vi "Notebook.vi"() -> ()   [LabVIEW 2019, in "Notebook.lvlib"]
uses:
  Notebook.lvlib
  System.Windows.Forms
  Notebook Action Q Element.ctl
  Notebook Action List.ctl
  System.Drawing
  Rich Text Box/Text Colors.ctl
  Rich Text Box/Formatted Text.ctl
  Rich Text Box/Text Formatting.ctl
  Notebook Saved Global.vi
  Rich Text Box/Rich Text Box.lvlib
  Variant/Variant to Data/Variant to Data.lvlib
panel:
  in  "Notebook Content":refnum<k24>(container)
types:
  T1 = enum32{"Invalid", "Standard", "Closed", "Hidden", "Minimized", "Maximized"}
  T2 = typedef "Notebook.lvlib/Notebook Action Q Element.ctl" = cluster{"Action":T3, "Variant":variant}
  T3 = typedef "Notebook.lvlib/Notebook Action List.ctl" = enum16{"Idle", "Init", "Check Content Change", "User added content", "Program added text", "Program added Picture ", "Save Notebook", "Quit", "Open", "Close", "Update Window Title"}
  T4 = typedef "Rich Text Box.lvlib/Text Colors.ctl" = enum16{"Unchanged", "Black", "Blue", "Gray", "Green", "Red", "White"}
  T5 = typedef "Rich Text Box.lvlib/Formatted Text.ctl" = cluster{"Text":string, "Text Formatting":T6}
  T6 = typedef "Rich Text Box.lvlib/Text Formatting.ctl" = cluster{"Font":string, "Text Color":T4, "Text Background Color":T4, "Text Style":enum16{"Regular", "Bold", "Italic", "Underline", "Strikeout"}, "Font Size (Points)":dbl, "Text Alignment":i32}
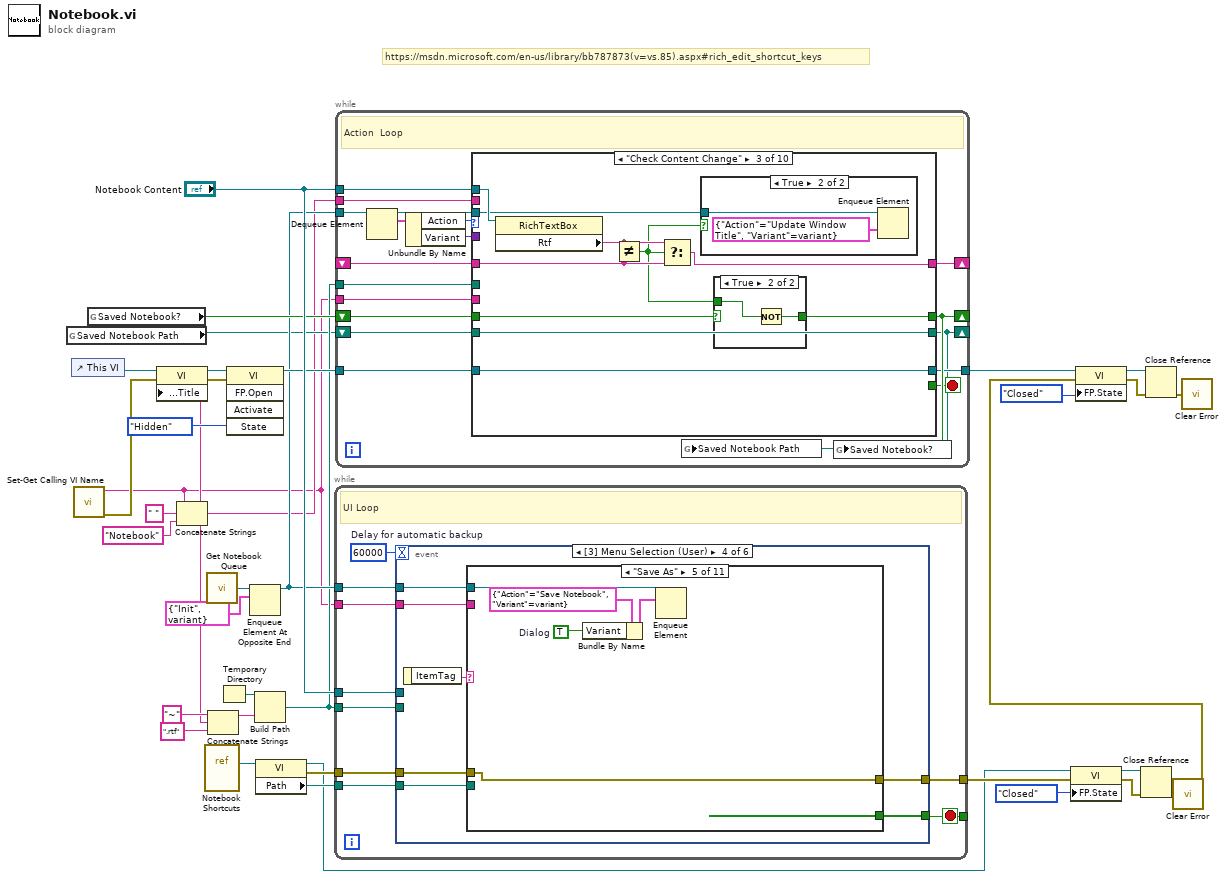
[diagram p0: block diagram]
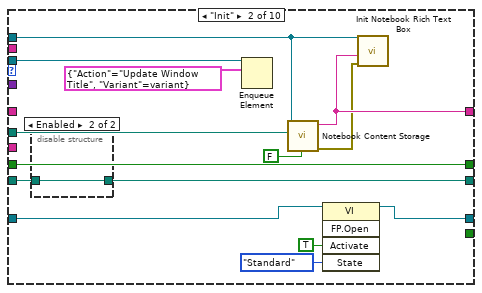
[diagram p3: hidden frame]
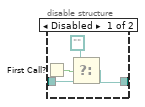
[diagram p4: hidden frame]
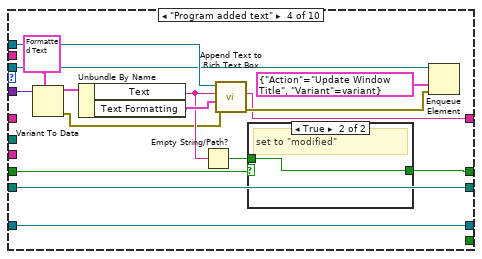
[diagram p7: hidden frame]
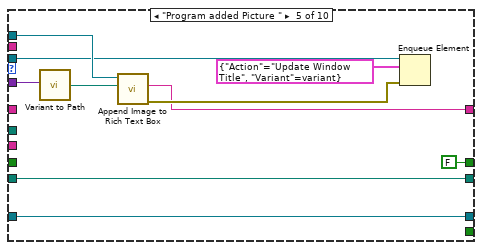
[diagram p9: hidden frame]
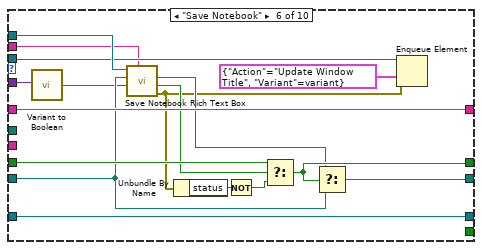
[diagram p10: hidden frame]
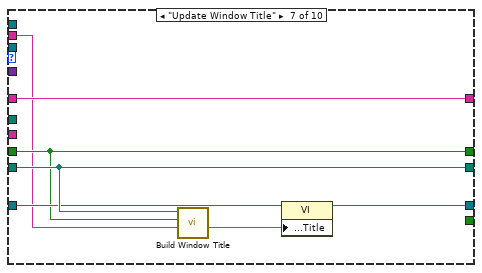
[diagram p11: hidden frame]
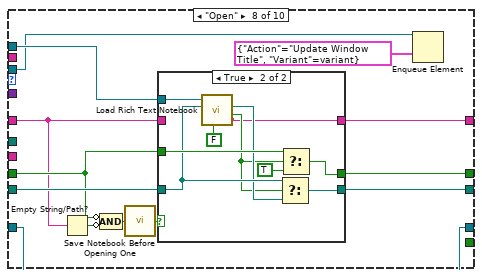
[diagram p12: hidden frame]
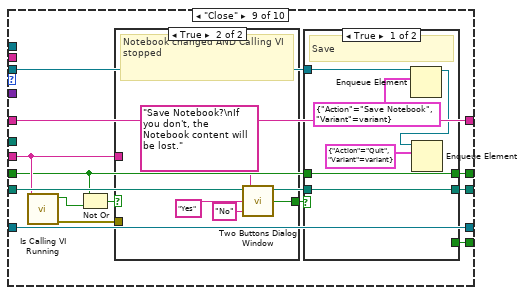
[diagram p14: hidden frame]
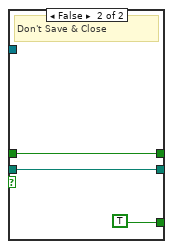
[diagram p15: hidden frame]
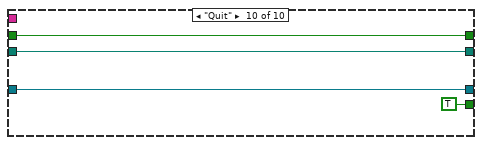
[diagram p17: hidden frame]
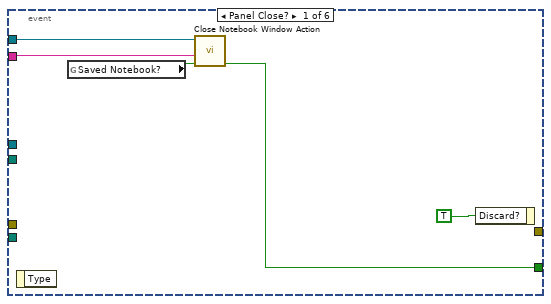
[diagram p18: hidden frame]
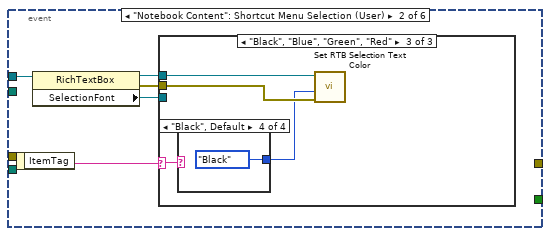
[diagram p19: hidden frame]
diagram:
  # "https://msdn.microsoft.com/en-us/library/bb787873(v=vs.85).aspx#rich_edit_shortcut_keys"
  n1 = global read "Notebook Saved Global.vi" "Saved Notebook Path"() -> (w17:path)
  n2 = control-ref of="This VI"() -> (w31:refnum<vi>)
  n3 = call "Set-Get Calling VI Name.vi"() -> ("Error Out"=w3:errorcluster, "Calling VI Name"=w1:string)  [unwired: 10 in]
  n4 = global read "Notebook Saved Global.vi" "Saved Notebook?"() -> (w28:bool)
  n5 = Concatenate Strings(w1, " " ("string"), "Notebook" ("string")) -> (w2:string)
  n6 = property class="VI"(reference=w31, error in=w3, "Front Panel.Title"=w2) -> (reference out=w25:refnum<vi>, error out=w16:errorcluster)
  n7 = vi-ref "Notebook Shortcuts.vi"() -> (w13:refnum<vi>)
  n8 = call "Get Notebook Queue.vi"() -> ("Notebook Queue"=w27:refnum<queue>)  [unwired: 9 in]
  n9 = Concatenate Strings("~" ("string"), w2, ".rtf" ("format string")) -> (w19:string)
  n10 = Temporary Directory() -> (w32:path)
  n11 = invoke class="VI" method="FP.Open"(reference=w25, error in=w16, "State"=T1."Hidden") -> (reference out=w30:refnum<vi>)  [unwired: 2 in, 4 out]
  n12 = Enqueue Element At Opposite End(queue=w27, element=T2 {"Action"=enum."Init", "Variant"=variant}) -> (queue out=w26:refnum<queue>)  [unwired: 2 in, 2 out]
  n13 = Build Path(base path=w32, name or relative path=w19) -> (appended path=w18:path)
  n14 = property class="VI"(reference=w13) -> (reference out=w7:refnum<vi>, error out=w12:errorcluster, "Path"=w11:path)  [unwired: 1 in]
  n15 = while {
    tunnel: w26 -> [w45]
    tunnel: "Notebook Content" -> [w43]
    tunnel: w1 -> [w41]
    tunnel: w18 -> [w42]
    tunnel: w12 -> [w40]
    tunnel: w11 -> [w39]
    tunnel: [w38] -> _
    tunnel: [w37] -> w8
    stop <- w38 stop-if-true
    w44 = 60000  # Delay for automatic backup
    # "UI Loop"
    n16 = event shown="[3] Menu Selection (User)" {
      selector: _ -> [_ _ _ _ _ _]
      dyn-events: _ -> [_ _ _ _ _ _]
      timeout: w44 -> [_ _ _ _ _ _]
      tunnel: [w49 _ _ w88 w129 _] -> w38
      tunnel: w45 -> [w50 _ w83 w89 w130 _]
      tunnel: w43 -> [_ w54 w81 _ _ w143]
      tunnel: w42 -> [_ _ w80 _ _ _]
      tunnel: w41 -> [w46 _ _ w87 w128 _]
      tunnel: w40 -> [_ _ _ w86 _ _]
      tunnel: w39 -> [_ _ _ w85 _ _]
      tunnel: [_ _ _ w84 _ _] -> w37
      event Panel Close? {
        n17 = event-data() -> ()  [unwired: 1 in, 1 out]
        n18 = global read "Notebook Saved Global.vi" "Saved Notebook?"() -> (w47:bool)
        n19 = call "Close Notebook Window Action.vi"("Notebook Saved?"=w47, "Main VI Name"=w46, "Notebook Queue"=w50) -> ("Quit?"=w49:bool)  [unwired: 8 in]
        n20 = event-data("Discard?"=TRUE) -> ()  [unwired: 1 in, 1 out]
      }
      event "Notebook Content": Shortcut Menu Selection (User) {
        n21 = event-data() -> ("ItemTag"=w55:string)  [unwired: 1 in]
        n22 = property class="RichTextBox"(reference=w54) -> (reference out=w51:refnum<k24>, error out=w52:errorcluster, "SelectionFont"=w53:refnum<k24>)  [unwired: 1 in]
        n23 = case shown="\"Black\", \"Blue\", \"Green\", \"Red\"" w55 {
          selector: w55 -> [_ w61 w72]
          tunnel: w53 -> [_ w65 _]
          tunnel: w52 -> [_ w60 w73]
          tunnel: w51 -> [_ w57 w74]
          frame "", Default {
          }
          frame "Bold", "Italic", "Regular", "Strikeout", "Underline" {
            n24 = property class="Font"(reference=w65, error in=w60) -> (error out=w59:errorcluster, "Name"=w64:string, "SizeInPoints"=w63:sgl)  [unwired: 1 out]
            n25 = case shown="\"Bold\"" w61 {
              tunnel: [w66 w67 w68 w69 w70] -> w62
              frame "Regular", Default {
                w66 = 0 items=["Regular"=0, "Bold"=1, "Italic"=2, "Underline"=4, "Strikeout"=8] ("style")
              }
              frame "Bold" {
                w67 = 1 items=["Regular"=0, "Bold"=1, "Italic"=2, "Underline"=4, "Strikeout"=8] ("style")
              }
              frame "Italic" {
                w68 = 2 items=["Regular"=0, "Bold"=1, "Italic"=2, "Underline"=4, "Strikeout"=8] ("style")
              }
              frame "Underline" {
                w69 = 4 items=["Regular"=0, "Bold"=1, "Italic"=2, "Underline"=4, "Strikeout"=8] ("style")
              }
              frame "Strikeout" {
                w70 = 8 items=["Regular"=0, "Bold"=1, "Italic"=2, "Underline"=4, "Strikeout"=8] ("style")
              }
            }
            n26 = constructor class="Font"(error in=w59, "familyName"=w64, "emSize"=w63, "unit"=w62) -> (reference out=w56:refnum<k24>, error out=w58:errorcluster)  [unwired: 2 in, 4 out]
            n27 = property class="RichTextBox"(reference=w57, error in=w58, "SelectionFont"=w56) -> ()  [unwired: 2 out]
          }
          frame "Black", "Blue", "Green", "Red" {
            n28 = case shown="\"Black\", Default" w72 {
              tunnel: [Text_Colors."Blue" ("Text Color") Text_Colors."Green" ("Text Color") Text_Colors."Red" ("Text Color") Text_Colors."Black" ("Text Color")] -> w71
              frame "Blue" {
              }
              frame "Green" {
              }
              frame "Red" {
              }
              frame "Black", Default {
              }
            }
            n29 = call "Set RTB Selection Text Color.vi"("Error In"=w73, "Text Color"=w71, ".NET RTB Refnum in"=w74) -> ()  [unwired: 7 in, 2 out]
          }
        }
      }
      event Timeout {
        n30 = event-data() -> ()  [unwired: 1 in, 1 out]
        n31 = call "Notebook Content Storage.vi"("Save(T)/Load(F)"=TRUE, "path"=w80, ".NET Refnum in"=w81) -> ()  [unwired: 7 in, 2 out]
        n32 = Enqueue Element(queue=w83, element=T2 {"Action"=enum."Check Content Change", "Variant"=variant}) -> ()  [unwired: 2 in, 3 out]
      }
      event Menu Selection (User) {
        n33 = event-data() -> ("ItemTag"=w90:string)  [unwired: 1 in]
        n34 = case shown="\"Save As\"" w90 {
          tunnel: w89 -> [_ _ w95 w100 w105 w110 _ w122 _ _ _]
          tunnel: [_ _ _ _ _ w109 _ _ _ _ _] -> w88
          tunnel: w87 -> [_ _ _ _ _ w107 _ _ _ _ _]
          tunnel: w86 -> [w91 w92 w93 w96 w101 w106 w111 w112 w123 w124 w126]
          tunnel: w85 -> [_ _ _ _ _ _ _ _ _ _ w127]
          tunnel: [w91 w92 w93 w96 w101 w106 w111 w112 w123 w124 w125] -> w84
          frame "", Default {
          }
          frame "---------File----------" {
          }
          frame "Open" {
            n35 = Enqueue Element(queue=w95, element=T2 {"Action"=enum."Open", "Variant"=variant}) -> ()  [unwired: 2 in, 3 out]
          }
          frame "Save" {
            w97 = FALSE  # No dialog
            n36 = Bundle By Name(cluster=T2 {"Action"=enum."Save Notebook", "Variant"=variant} ("element"), "Variant"=w97) -> (w98:T2)
            n37 = Enqueue Element(queue=w100, element=w98) -> ()  [unwired: 2 in, 3 out]
          }
          frame "Save As" {
            w102 = TRUE  # Dialog
            n38 = Bundle By Name(cluster=T2 {"Action"=enum."Save Notebook", "Variant"=variant} ("element"), "Variant"=w102) -> (w103:T2)
            n39 = Enqueue Element(queue=w105, element=w103) -> ()  [unwired: 2 in, 3 out]
          }
          frame "Close" {
            n40 = global read "Notebook Saved Global.vi" "Saved Notebook?"() -> (w108:bool)
            n41 = call "Close Notebook Window Action.vi"("Notebook Saved?"=w108, "Main VI Name"=w107, "Notebook Queue"=w110) -> ("Quit?"=w109:bool)  [unwired: 8 in]
          }
          frame "----------Edit----------" {
          }
          frame "Paste Current Date & Time" {
            n42 = call "Current Date & Time String.vi"() -> ("time string"=w113:string, "date string"=w114:string)  [unwired: 9 in, 1 out]
            n43 = Format Into String(format string="Current Date & Time: %s, %s" ("initial string"), w114, w113) -> (resulting string=w117:string)  [unwired: 2 in, 1 out]
            n44 = call "Message Style.vi"() -> ("Message Formatting"=w116:T6)
            n45 = Bundle By Name(cluster=T5 {"Text"="", "Text Formatting"={"Font"="Default", "Text Color"=enum."Unchanged", "Text Background Color"=enum."Unchanged", "Text Style"=enum."Regular", "Font Size (Points)"=-1.0, "Text Alignment"=0}} ("Formatted Text"), "Text"=w117, "Text Formatting"=w116) -> (w118:T5)
            n46 = Bundle By Name(cluster=T2 {"Action"=enum."Program added text", "Variant"=variant} ("element"), "Variant"=w118) -> (w120:T2)
            n47 = Enqueue Element(queue=w122, element=w120) -> ()  [unwired: 2 in, 3 out]
          }
          frame "Find..." {
          }
          frame "-------- Help ---------" {
          }
          frame "Show Notebook Shortcuts" {
            n48 = call "Run Vi.vi"("VI Path"=w127, "error in (no error)"=w126) -> ("error out"=w125:errorcluster)  [unwired: 6 in, 1 out]
          }
        }
      }
      event "Notebook Content": Shortcut Menu Selection (App) {
        n49 = event-data() -> ("ItemTag"=w131:string)  [unwired: 1 in, 1 out]
        n50 = case shown="\"Paste Current Date & Time\"" w131 {
          tunnel: w130 -> [_ w142]
          tunnel: [_ FALSE ("Quit?")] -> w129
          tunnel: w128 -> [_ _]
          frame "", Default {
          }
          frame "Paste Current Date & Time" {
            n51 = call "Current Date & Time String.vi"() -> ("time string"=w134:string, "date string"=w133:string)  [unwired: 9 in, 1 out]
            n52 = Format Into String(format string="Current Date & Time: %s, %s" ("initial string"), w133, w134) -> (resulting string=w137:string)  [unwired: 2 in, 1 out]
            n53 = call "Message Style.vi"() -> ("Message Formatting"=w136:T6)
            n54 = Bundle By Name(cluster=T5 {"Text"="", "Text Formatting"={"Font"="Default", "Text Color"=enum."Unchanged", "Text Background Color"=enum."Unchanged", "Text Style"=enum."Regular", "Font Size (Points)"=-1.0, "Text Alignment"=0}} ("Formatted Text"), "Text"=w137, "Text Formatting"=w136) -> (w138:T5)
            n55 = Bundle By Name(cluster=T2 {"Action"=enum."Program added text", "Variant"=variant} ("element"), "Variant"=w138) -> (w140:T2)
            n56 = Enqueue Element(queue=w142, element=w140) -> ()  [unwired: 2 in, 3 out]
          }
        }
      }
      event Panel Resize {
        n57 = event-data() -> ()  [unwired: 1 in, 1 out]
        n58 = disable-structure shown="Enabled" {
          disable-tunnel: w143 -> [_ w145]
          frame Disabled {
            w144 = inf
          }
          frame Enabled {
            n59 = invoke class="RichTextBox" method="ScrollToCaret"(reference=w145) -> ()  [unwired: 2 in, 3 out]
          }
        }
      }
    }
  }
  n60 = while {
    tunnel: w26 -> [w163]
    shift-right: [w156] -> _
    shift-left: w28 -> [w160]
    shift-right: [w147] -> _
    shift-left: w17 -> [w159]
    tunnel: w30 -> [w153]
    tunnel: [w151] -> w36
    tunnel: "Notebook Content" -> [w155]
    tunnel: w1 -> [w152]
    shift-right: [w150] -> _
    shift-left: _ -> [w149]
    tunnel: w18 -> [w148]
    tunnel: w2 -> [w146]
    stop <- w154 stop-if-true
    # "Action  Loop"
    n61 = Dequeue Element(queue=w163) -> (queue out=w158:refnum<queue>, element=w162:T2)  [unwired: 2 in, 2 out]
    n62 = Unbundle By Name(w162) -> ("Action"=w161:T3, "Variant"=w157:variant)
    n63 = case shown="\"Check Content Change\"" w161 {
      tunnel: w160 -> [w167 w168 w189 w204 _ w242 w249 w263 w282 w310]
      tunnel: [w167 w168 w188 w203 FALSE ("Saved?") w237 w249 w264 w291 w310] -> w156
      tunnel: w159 -> [w166 w178 w196 w217 w229 w239 w253 w266 w289 w309]
      tunnel: [w166 w177 w196 w217 w229 w240 w253 w265 w288 w309] -> w147
      tunnel: w158 -> [_ w170 w190 w206 w222 w236 _ w256 w290 _]
      tunnel: w157 -> [_ _ _ w215 w227 w234 _ _ _ _]
      tunnel: w155 -> [_ w172 w194 w216 w228 w246 _ w259 _ _]
      tunnel: [_ _ _ _ _ _ _ _ w287 TRUE] -> w154
      tunnel: w153 -> [w165 w181 w195 w209 w224 w243 w251 w258 w286 w307]
      tunnel: w152 -> [_ _ _ _ _ _ _ _ w284 _]
      tunnel: [w165 w176 w195 w209 w224 w243 w250 w258 w286 w307] -> w151
      tunnel: [w164 w175 w191 w205 w220 w241 w248 w255 w285 _] -> w150
      tunnel: w149 -> [w164 _ w192 _ _ w241 w248 w254 w285 _]
      tunnel: w148 -> [_ w173 _ _ _ _ _ _ _ _]
      tunnel: w146 -> [_ _ _ _ _ w230 w247 _ _ _]
      frame "Idle", Default {
      }
      frame "Init" {
        n64 = disable-structure shown="Enabled" {
          disable-tunnel: w178 -> [w185 w186]
          disable-tunnel: [w184 w186] -> w177
          frame Disabled {
            n65 = First Call?() -> (First Call?: T/F=w182:bool)
            n66 = Select(t=path "", s=w182, f=w185) -> (s? t:f=w184:path)
          }
          frame Enabled {
          }
        }
        n67 = Enqueue Element(queue=w170, element=T2 {"Action"=enum."Update Window Title", "Variant"=variant}) -> ()  [unwired: 2 in, 3 out]
        n68 = call "Notebook Content Storage.vi"("Save(T)/Load(F)"=FALSE ("Set(T)/Get(F)"), "path"=w173, ".NET Refnum in"=w172) -> ("Error Out"=w171:errorcluster, "RTF content"=w175:string)  [unwired: 7 in]
        n69 = invoke class="VI" method="FP.Open"(reference=w181, "Activate"=TRUE ("Activate?"), "State"=T1."Standard") -> (reference out=w176:refnum<vi>)  [unwired: 2 in, 4 out]
        n70 = call "Init Notebook Rich Text Box.vi"("Error In"=w171, "Notebook Content"=w175, ".NET Refnum in"=w172) -> ()  [unwired: 8 in, 1 out]
      }
      frame "Check Content Change" {
        n71 = property class="RichTextBox"(reference=w194) -> ("Rtf"=w193:string)  [unwired: 1 in, 2 out]
        n72 = Not Equal?(x=w193, y=w192) -> (x != y?=w187:bool)
        n73 = Select(t=w193, s=w187, f=w192) -> (s? t:f=w191:string)
        n74 = case shown="True" w187 {
          tunnel: w190 -> [_ w201]
          frame False {
          }
          frame True {
            n75 = Enqueue Element(queue=w201, element=T2 {"Action"=enum."Update Window Title", "Variant"=variant}) -> ()  [unwired: 2 in, 3 out]
          }
        }
        n76 = case shown="True" w189 {
          selector: w189 -> [w197 _]
          tunnel: [w197 w198] -> w188
          tunnel: w187 -> [_ w199]
          frame False {
          }
          frame True {
            n77 = Not(x=w199) -> (.not. x?=w198:bool)
          }
        }
      }
      frame "Program added text" {
        n78 = Variant To Data(type=T5 {"Text"="", "Text Formatting"={"Font"="Default", "Text Color"=enum."Unchanged", "Text Background Color"=enum."Unchanged", "Text Style"=enum."Regular", "Font Size (Points)"=-1.0, "Text Alignment"=0}} ("Formatted Text"), Variant=w215) -> (data=w213:T5, error out=w210:errorcluster)  [unwired: 1 in]
        n79 = Unbundle By Name(w213) -> ("Text"=w211:string, "Text Formatting"=w212:T6)
        n80 = Empty String/Path?(string/path=w211) -> (empty?=w202:bool)
        n81 = call "Append Text to Rich Text Box.vi"("error in (no error)"=w210, "Text Formatting"=w212, "String"=w211, ".NET Refnum in"=w216) -> ("Error Out"=w207:errorcluster, "Rtf Content"=w205:string)  [unwired: 6 in]
        n82 = case shown="True" w204 {
          selector: w204 -> [w218 _]
          tunnel: [w218 w219] -> w203
          tunnel: w202 -> [_ w219]
          frame False {
            # "remains \"modified\""
          }
          frame True {
            # "set to \"modified\""
          }
        }
        n83 = Enqueue Element(queue=w206, element=T2 {"Action"=enum."Update Window Title", "Variant"=variant}, error in (no error)=w207) -> ()  [unwired: 1 in, 3 out]
      }
      frame "Program added Picture " {
        n84 = call "Variant to Path.vi"("Variant"=w227) -> ("Path"=w226:path)  [unwired: 8 in]
        n85 = call "Append Image to Rich Text Box.vi"("Image File Path"=w226, ".NET Refnum in"=w228) -> ("error out"=w221:errorcluster, "Rtf Content"=w220:string)  [unwired: 8 in]
        n86 = Enqueue Element(queue=w222, element=T2 {"Action"=enum."Update Window Title", "Variant"=variant}, error in (no error)=w221) -> ()  [unwired: 1 in, 3 out]
      }
      frame "Save Notebook" {
        n87 = call "Variant to Boolean.vi"("Variant"=w234) -> ("Value"=w233:bool)  [unwired: 8 in]
        n88 = call "Save Notebook Rich Text Box.vi"("Default Notebook File Name (Notebook)"=w230, "Dialog (F)"=w233, "File Path Control"=w239, ".NET Refnum in"=w246) -> ("Error Out"=w231:errorcluster, "cancelled"=w238:bool, "File Path out"=w232:path)  [unwired: 5 in]
        n89 = Unbundle By Name(w231) -> ("status"=w245:bool)
        n90 = Not(x=w245) -> (.not. x?=w244:bool)
        n91 = Select(t=w242, s=w238, f=w244) -> (s? t:f=w237:bool)
        n92 = Select(t=w232, s=w237, f=w239) -> (s? t:f=w240:path)
        n93 = Enqueue Element(queue=w236, element=T2 {"Action"=enum."Update Window Title", "Variant"=variant}, error in (no error)=w231) -> ()  [unwired: 1 in, 3 out]
      }
      frame "Update Window Title" {
        n94 = call "Build Window Title.vi"("Root Window Title"=w247, "Saved Notebook?"=w249, "File Path in"=w253) -> ("Modified Window Title"=w252:string)  [unwired: 8 in]
        n95 = property class="VI"(reference=w251, "Front Panel.Title"=w252) -> (reference out=w250:refnum<vi>)  [unwired: 1 in, 1 out]
      }
      frame "Open" {
        n96 = Empty String/Path?(string/path=w254) -> (empty?=w260:bool)
        n97 = Compound Arithmetic op=AND(invert w263, invert w260) -> (w262:bool)
        n98 = call "Save Notebook Before Opening One.vi"("Not saved?"=w262) -> ("Save?"=w261:bool)  [unwired: 8 in]
        n99 = case shown="True" w261 {
          tunnel: w266 -> [w268 w277]
          tunnel: [w268 w276] -> w265
          tunnel: [w269 w279] -> w264
          tunnel: w263 -> [w269 w278]
          tunnel: w259 -> [_ w275]
          tunnel: [w267 w271] -> w255
          tunnel: w254 -> [w267 _]
          frame False {
          }
          frame True {
            n100 = call "Load Rich Text Notebook.vi"("Backup?"=FALSE, "File Path Control"=w277, ".NET Refnum in"=w275) -> ("cancelled"=w273:bool, "File Path out"=w274:path, "RTF content"=w271:string)  [unwired: 4 in, 2 out]
            n101 = Select(t=w277, s=w273, f=w274) -> (s? t:f=w276:path)
            n102 = Select(t=w278, s=w273, f=TRUE) -> (s? t:f=w279:bool)
          }
        }
        n103 = Enqueue Element(queue=w256, element=T2 {"Action"=enum."Update Window Title", "Variant"=variant}) -> ()  [unwired: 2 in, 3 out]
      }
      frame "Close" {
        n104 = call "Is Calling VI Running.vi"("Calling VI Name"=w284) -> ("Error Out"=w280:errorcluster, "Running?"=w283:bool)  [unwired: 9 in]
        n105 = Not Or(1:w283, 2:w282) -> (0:w281:bool)
        n106 = case shown="True" w281 {
          selector: w281 -> [w302 _]
          tunnel: [w302 w305] -> w292
          tunnel: w284 -> [_ _]
          tunnel: w280 -> [_ _]
          frame False {
            # "Notebook unchanged OR Calling VI still running"
          }
          frame True {
            # "Notebook changed AND Calling VI stopped"
            n107 = call "Two Buttons Dialog Window.vi"("Cancel Button Text"="No" ("F button name (\"Cancel\")"), "OK Button Text"="Yes" ("T button name (\"OK\")"), "Message"="Save Notebook?\nIf you don't, the Notebook content will be lost." ("message")) -> ("OK?"=w305:bool)
          }
        }
        n108 = case shown="True" w292 {
          tunnel: w282 -> [w296 w299]
          tunnel: [w296 w299] -> w291
          tunnel: w290 -> [w298 _]
          tunnel: w289 -> [w295 w301]
          tunnel: [w295 w301] -> w288
          tunnel: [_ TRUE] -> w287
          frame True {
            # "Save"
            n109 = Enqueue Element(queue=w298, element=T2 {"Action"=enum."Save Notebook", "Variant"=variant}) -> (queue out=w293:refnum<queue>)  [unwired: 2 in, 2 out]
            n110 = Enqueue Element(queue=w293, element=T2 {"Action"=enum."Quit", "Variant"=variant}) -> ()  [unwired: 2 in, 3 out]
          }
          frame False {
            # "Don't Save & Close"
          }
        }
      }
      frame "Quit" {
      }
    }
    n111 = global write "Notebook Saved Global.vi" "Saved Notebook Path"(w147) -> ()
    n112 = global write "Notebook Saved Global.vi" "Saved Notebook?"(w156) -> ()
  }
  n113 = property class="VI"(reference=w7, error in=w8, "FP.State"=T1."Closed" ("Front Panel Window:State")) -> (reference out=w9:refnum<vi>, error out=w10:errorcluster)
  n114 = Close Reference(reference=w9, error in (no error)=w10) -> (error out=w5:errorcluster)
  n115 = call "Clear Error.vi"("Error In"=w5) -> ("no Error Out"=w4:errorcluster)  [unwired: 8 in]
  n116 = property class="VI"(reference=w36, error in=w4, "FP.State"=T1."Closed" ("Front Panel Window:State")) -> (reference out=w34:refnum<vi>, error out=w15:errorcluster)
  n117 = Close Reference(reference=w34, error in (no error)=w15) -> (error out=w14:errorcluster)
  n118 = call "Clear Error.vi"("Error In"=w14) -> ()  [unwired: 8 in, 1 out]
